vi "Database Open Connection.vi"(8 "error in":errorcluster, 11 "Database File Path":path) -> (0 "error out":errorcluster, 3 "valid URL":string)   [LabVIEW 2015, in "DatabaseAPI.lvclass"]
uses:
  DatabaseAPI.lvclass
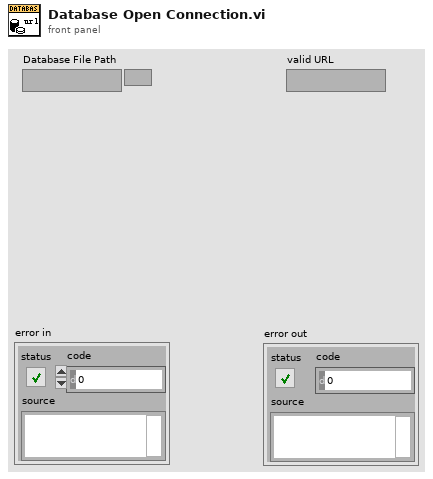
[diagram p1: front panel]
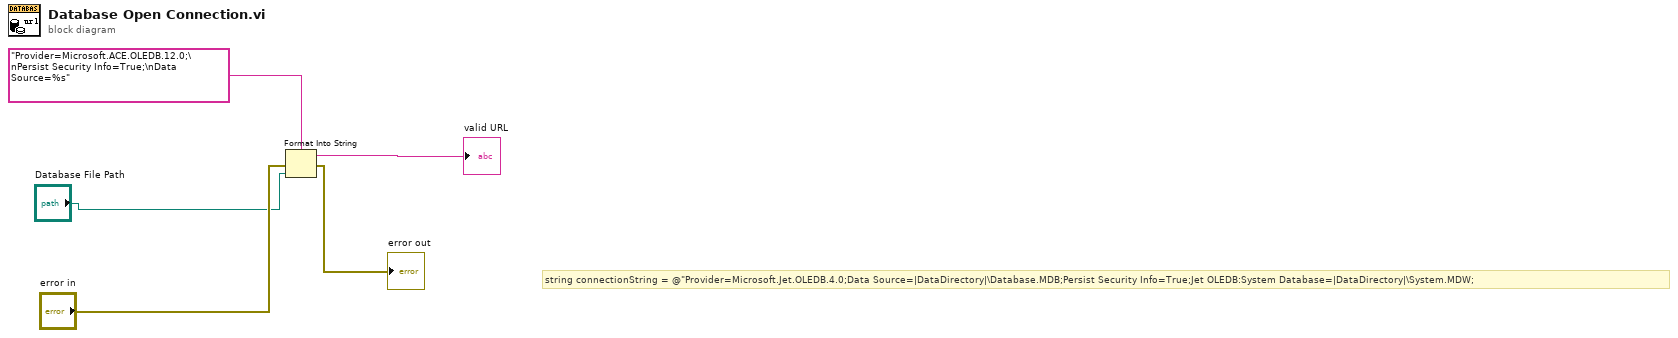
[diagram p0: block diagram]
diagram:
  # "string connectionString = @\"Provider=Microsoft.Jet.OLEDB.4.0;Data Source=|DataDirectory|\\Database.MDB;Persist Security Info=True;Jet OLEDB:System Database=|DataDirectory|\\System.MDW;"
  n1 = Format Into String(format string="Provider=Microsoft.ACE.OLEDB.12.0;\nPersist Security Info=True;\nData Source=%s", error in="error in", "Database File Path") -> (resulting string=→"valid URL":string, error out=→"error out":errorcluster)  [unwired: 1 in]
